vi "Send Message And Grep Response.vi"(0 "VISA resource name":refnum<visa-resource-name>, 5 "Command (\"\")":string, 7 "Strings (\"\")":string, 11 "error in (no error)":errorcluster, 14 "Source (\"\")":string) -> (4 "VISA resource name out":refnum<visa-resource-name>, 6 "Output Strings":string, 8 "Result":bool, 15 "error out":errorcluster)   [LabVIEW 2020, in "Yokogawa GX Series.lvlib"]
doc: "This VI sets the alarm hysteresis for <B>DX1000/DX2000 series</B>.\nThis VI can be used on Basic Setting Mode at the <B>Set Execution Mode.VI</B>.\n\nAlarm settings on computation channels can be specified on models with the /M1 or /PM1 math option.\nAlarm settings on external input channels can be specified on models with the /MC1 external input channel option."
uses:
  <instrlib>/Yokogawa GX Series/Yokogawa GX Series.lvlib
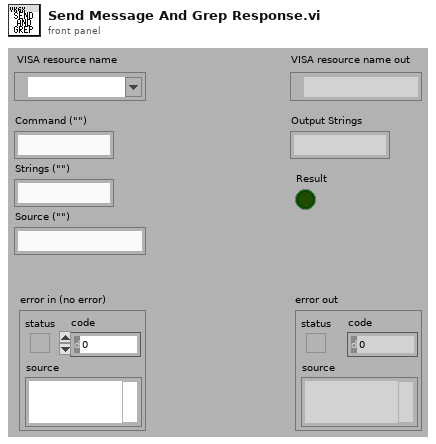
[diagram p1: front panel]
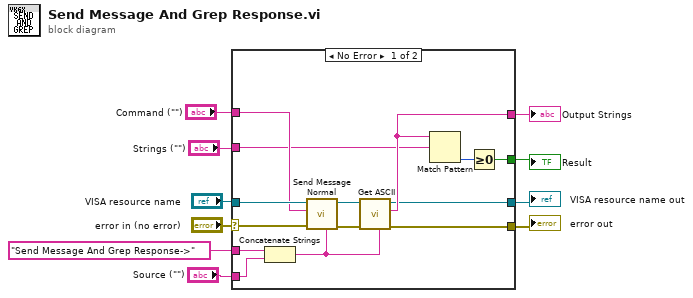
[diagram p0: block diagram]
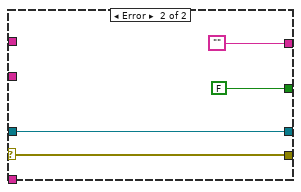
[diagram p2: hidden frame]
diagram:
  n1 = case shown="No Error" "error in (no error)" {
    selector: "error in (no error)" -> [w23 w27]
    tunnel: "VISA resource name" -> [w24 w28]
    tunnel: "Command (\"\")" -> [w22 _]
    tunnel: "Strings (\"\")" -> [w18 _]
    tunnel: [w19 ""] -> w7
    tunnel: [w17 w27] -> w6
    tunnel: [w16 w28] -> w5
    tunnel: [w14 FALSE] -> w4
    tunnel: "Source (\"\")" -> [w12 _]
    tunnel: "Send Message And Grep Response->" -> [w13 _]
    frame No Error {
      n2 = Concatenate Strings(w13, w12) -> (w11:string)
      n3 = call <instrlib>:"Send Message Normal.vi"("Source (\"\")"=w11, "error in (no error)"=w23, "Send Message (\"\")"=w22, "VISA resource name"=w24) -> ("error out"=w21:errorcluster, "VISA resource name out"=w20:refnum<visa-resource-name>)  [unwired: 5 in, 1 out]
      n4 = call <instrlib>:"Get ASCII.vi"("Source (\"\")"=w11, "error in (no error)"=w21, "VISA resource name"=w20) -> ("error out"=w17:errorcluster, "ASCII Data"=w19:string, "VISA resource name out"=w16:refnum<visa-resource-name>)  [unwired: 6 in]
      n5 = Match Pattern(string=w19, regular expression=w18) -> (offset past match=w15:i32)  [unwired: 1 in, 3 out]
      n6 = Greater Or Equal To 0?(x=w15) -> (x >= 0?=w14:bool)
    }
    frame Error {
    }
  }
  "error out" <- w6
  "VISA resource name out" <- w5
  "Output Strings" <- w7
  "Result" <- w4
